vi "Delete Application Data Directory.vi"(8 "error in":errorcluster) -> (0 "error out":errorcluster)   [LabVIEW 2020, in "SEECD System Explorer.lvlib"]
uses:
  SEECD System Explorer.lvlib
  <vilib>/Utility/sysdir.llb/Get System Directory.vi
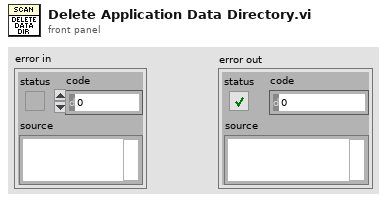
[diagram p1: front panel]
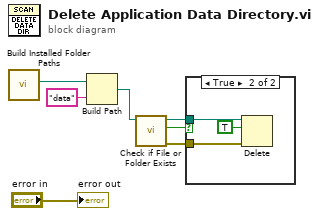
[diagram p0: block diagram]
diagram:
  n1 = call "Build Installed Folder Paths.vi"() -> ("Application Folder Path"=w5:path)  [unwired: 10 in, 1 out]
  n2 = Build Path(base path=w5, name or relative path="data") -> (appended path=w3:path)
  n3 = call <vilib>:"Check if File or Folder Exists.vi"("path"=w3) -> ("error out"=w7:errorcluster, "file or folder exists?"=w6:bool, "dup path"=w2:path)  [unwired: 8 in]
  n4 = case shown="True" w6 {
    tunnel: w7 -> [_ w9]
    tunnel: w2 -> [_ w10]
    frame False {
    }
    frame True {
      n5 = Delete(path (use dialog)=w10, entire hierarchy (F)=TRUE, error in=w9) -> ()  [unwired: 2 in, 3 out]
    }
  }
  "error out" <- "error in"
